vi "isTransitionRequested.vi"(11 "statemachine":refnum<class "statemachine.lvclass">) -> (2 "Transition Requested?":bool, 3 "statemachine":refnum<class "statemachine.lvclass">)   [LabVIEW 2020, in "eos.lvlib" / "statemachine.lvclass"]
uses:
  statemachine.lvclass
  statemachine.lvclass/statemachine.ctl
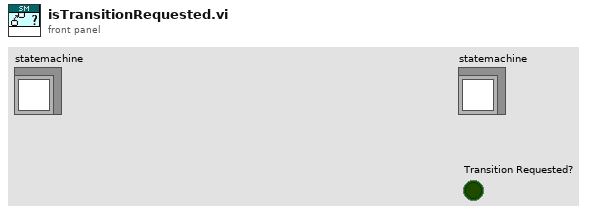
[diagram p1: front panel]
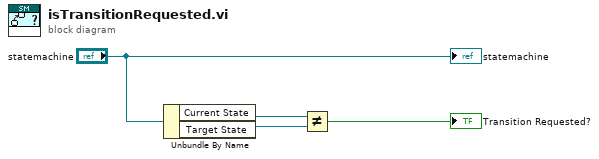
[diagram p0: block diagram]
diagram:
  n1 = Unbundle By Name("statemachine") -> ("Current State"=w2:refnum<class "state.lvclass">, "Target State"=w1:refnum<class "state.lvclass">)
  n2 = Not Equal?(x=w2, y=w1) -> (x != y?=→"Transition Requested?":bool)
  "statemachine" <- "statemachine"
